vi "kalman feedforward v onlyl.vi"(6 "ff vel?":bool, 7 "tick count":u32, 10 "state in":T1) -> (2 "state out":T1)   [LabVIEW 2010]
uses:
  integrating single axis kalman state.ctl
  <vilib>/rvi/FXPMathLib/FxpMul/XNode/nifxpmath_Multiplier.xnode
  <vilib>/rvi/FXPMathLib/FxpMul/subVIs/nifxpmath_Mul_SimConfig.ctl
  <vilib>/fxp/LVFixedPointQuantizationPolicyTypeDef.ctl
  <vilib>/fxp/LVFixedPointOverflowPolicyTypeDef.ctl
  <vilib>/rvi/FXPMathLib/FxpAdd/XNode/nifxpmath_Add.xnode
  <vilib>/rvi/FXPMathLib/FxpAdd/subVIs/nifxpmath_Add_SimConfig.ctl
  <vilib>/rvi/FXPMathLib/FxpMul/simVIs/DllFxpMulTemp_sub.vi
  <vilib>/rvi/FXPMathLib/FxpAdd/simVIs/DllFxpAddTemp_sub.vi
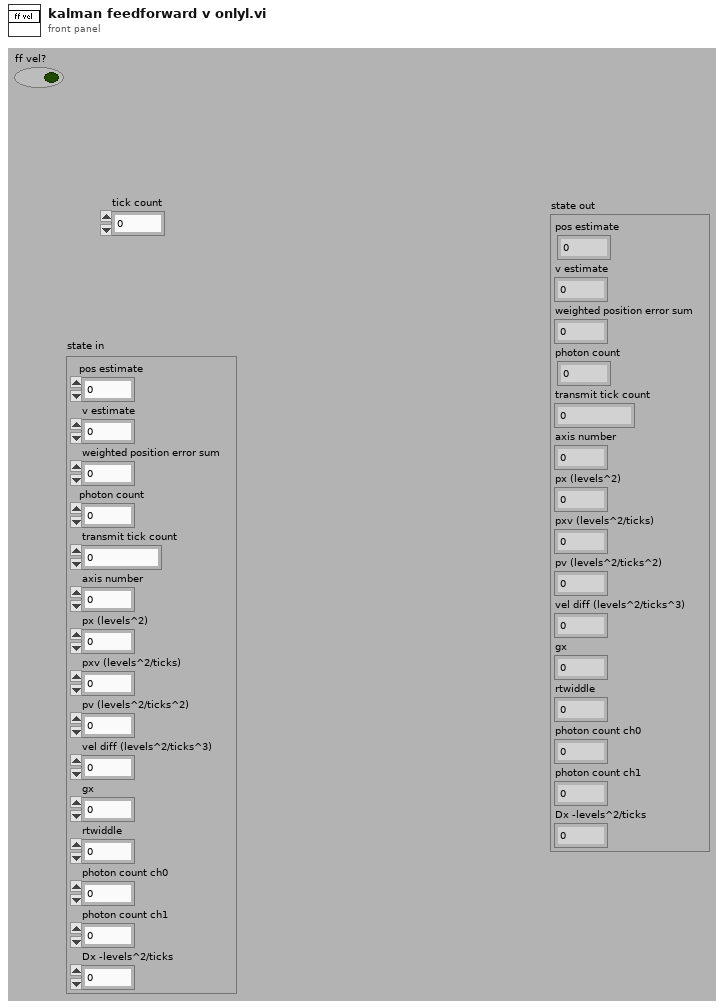
[diagram p1: front panel]
types:
  T1 = typedef "integrating single axis kalman state.ctl" = cluster{"pos estimate":fxp<+/-,32,16>, "v estimate":fxp<+/-,16,0>, "weighted position error sum":fxp<+/-,32,32>, "photon count":u32, "transmit tick count":u32, "axis number":u8, "px (levels^2)":fxp<+,32,19>, "pxv (levels^2/ticks)":fxp<+,32,2>, "pv (levels^2/ticks^2)":fxp<+,32,-14>, "vel diff (levels^2/ticks^3)":fxp<+,24,-22>, "gx":fxp<+,16,8>, "rtwiddle":fxp<+,16,26>, "photon count ch0":u32, "photon count ch1":u32, "Dx -levels^2/ticks":fxp<+,32,19>}
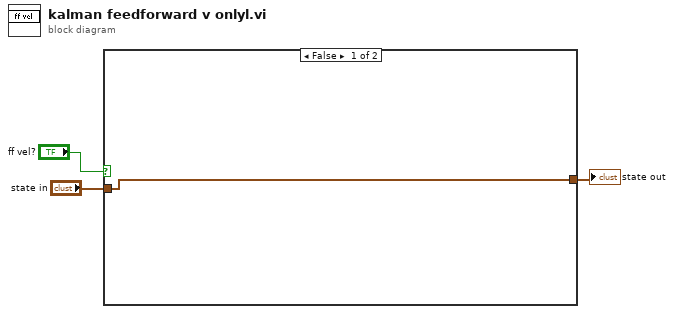
[diagram p0: block diagram]
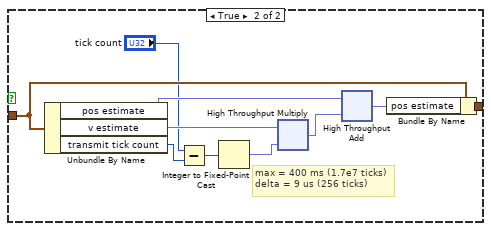
[diagram p2: hidden frame]
diagram:
  n1 = case shown="False" "ff vel?" {
    tunnel: "state in" -> [w4 w14]
    tunnel: [w4 w13] -> w2
    frame False {
    }
    frame True {
      # "max = 400 ms (1.7e7 ticks)\ndelta = 9 us (256 ticks)"
      n2 = Unbundle By Name(w14) -> ("pos estimate"=w11:fxp<+/-,32,16>, "v estimate"=w9:fxp<+/-,16,0>, "transmit tick count"=w6:u32)
      n3 = Subtract(x="tick count", y=w6) -> (x-y=w5:u32)
      n4 = Integer to Fixed-Point Cast(integer=w5) -> (fixed-point=w12:fxp<+,16,24>)  [unwired: 1 in]
      n5 = xnode "High Throughput Multiply"("x"=w9, "y"=w12) -> ("x*y"=w8:fxp<+/-,16,15>)
      n6 = xnode "High Throughput Add"("x"=w11, "y"=w8) -> ("x+y"=w10:fxp<+/-,32,16>)
      n7 = Bundle By Name(cluster=w14, "pos estimate"=w10) -> (w13:T1)
    }
  }
  "state out" <- w2
